vi "Field List Set Default.vi"(6 "FIELD (empty)":T2={"ixField"=0, "iSequenceOrder"=0, "sxFieldId"="", "sxSequenceId"="", "sDisplayName"="", "sValue"="", "sUnits"="", "nDataType"=enum."timestamp", "nNextItem"=enum."Reset", "fSystem"=FALSE, "fSystemValue"=FALSE, "fRequired"=FALSE, "fSetAtTest"=FALSE, "fTestField"=FALSE, "fDeleted"=FALSE, "fIndexed"=FALSE, "fFreeList"=FALSE}, 8 "error in (no error)":errorcluster, 9 "Default Value (\"\")":string, 10 "Flat List (\"\")":string, 11 "Connection Refnum":T1) -> (0 "error out":errorcluster, 2 "New Flat List":string, 3 "dup Connection Refnum":T1)   [LabVIEW 2011]
uses:
  Field Record.ctl
  Field DataTypes.ctl
  Field NextItem.ctl
  Summitek EXT/ODBC/SQL Controls/Connection Refnum.ctl
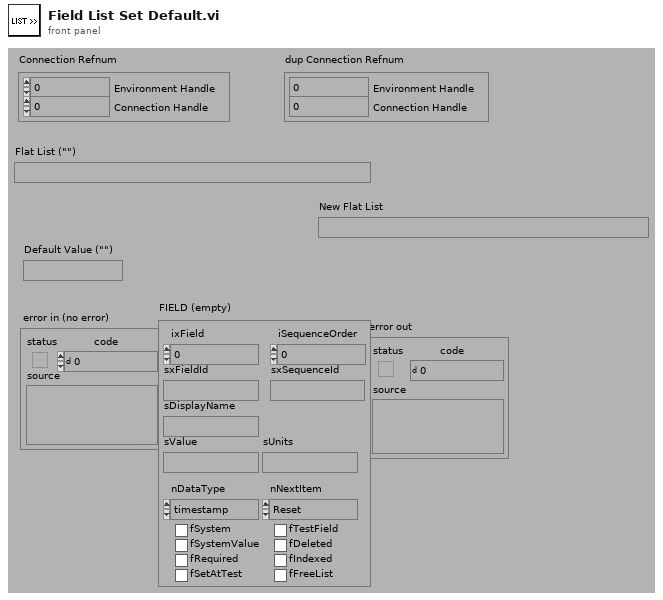
[diagram p1: front panel]
types:
  T1 = typedef "Connection Refnum.ctl" = cluster{"Environment Handle":i32, "Connection Handle":i32}
  T2 = typedef "Field Record.ctl" = cluster{"ixField":i32, "iSequenceOrder":i32, "sxFieldId":string, "sxSequenceId":string, "sDisplayName":string, "sValue":string, "sUnits":string, "nDataType":T3, "nNextItem":T4, "fSystem":bool, "fSystemValue":bool, "fRequired":bool, "fSetAtTest":bool, "fTestField":bool, "fDeleted":bool, "fIndexed":bool, "fFreeList":bool}
  T3 = typedef "Field DataTypes.ctl" = enum32{"text", "numeric", "list", "timestamp", "boolean"}
  T4 = typedef "Field NextItem.ctl" = enum32{"Reset", "Retain", "Auto-Increment"}
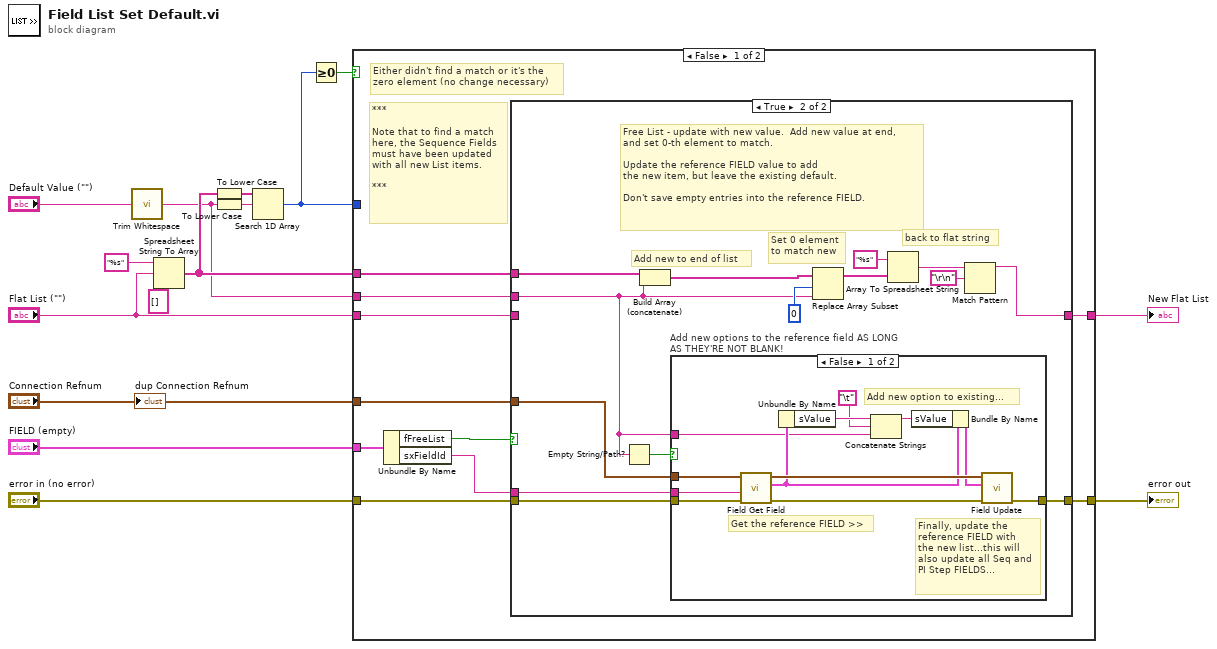
[diagram p0: block diagram]
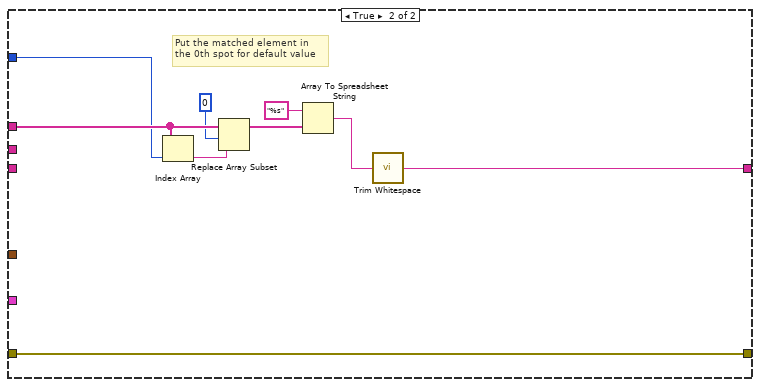
[diagram p4: hidden frame]
diagram:
  n1 = call <vilib>:"Trim Whitespace.vi"("string"="Default Value (\"\")") -> ("trimmed string"=w1:string)  [unwired: 1 in]
  n2 = Spreadsheet String To Array(format string="%s", spreadsheet string="Flat List (\"\")", array type (2D Dbl)=string[] []) -> (array=w7:string[])  [unwired: 1 out]
  n3 = To Lower Case(string=w7) -> (all lower case string=w13:string[])
  n4 = To Lower Case(string=w1) -> (all lower case string=w14:string)
  n5 = Search 1D Array(1D array=w13, element=w14) -> (index of element=w8:i32)  [unwired: 1 out]
  n6 = Greater Or Equal To 0?(x=w8) -> (x >= 0?=w9:bool)
  n7 = case shown="False" w9 {
    tunnel: "Flat List (\"\")" -> [w23 _]
    tunnel: [w22 w56] -> w10
    tunnel: w8 -> [_ w62]
    tunnel: w7 -> [w17 w63]
    tunnel: "Connection Refnum" -> [w20 _]
    tunnel: "FIELD (empty)" -> [w19 _]
    tunnel: "error in (no error)" -> [w25 w55]
    tunnel: [w24 w55] -> w3
    tunnel: w1 -> [w21 _]
    frame False {
      # "***\n\nNote that to find a match\nhere, the Sequence Fields\nmust have been updated\nwith all new List items.\n\n***"
      # "Either didn't find a match or it's the\nzero element (no change necessary)"
      n8 = Unbundle By Name(w19) -> ("fFreeList"=w16:bool, "sxFieldId"=w18:string)
      n9 = case shown="True" w16 {
        tunnel: w25 -> [w26 w40]
        tunnel: [w26 w41] -> w24
        tunnel: w23 -> [w27 _]
        tunnel: [w27 w28] -> w22
        tunnel: w21 -> [_ w32]
        tunnel: w20 -> [_ w39]
        tunnel: w18 -> [_ w38]
        tunnel: w17 -> [_ w36]
        frame False {
          # "Not a Free List - cannot update"
        }
        frame True {
          # "back to flat string"
          # "Set 0 element\nto match new"
          # "Add new to end of list"
          # "Free List - update with new value.  Add new value at end,\nand set 0-th element to match.\n\nUpdate the reference FIELD value to add\nthe new item, but leave the existing default.\n\nDon't save empty entries into the reference FIELD."
          n10 = Empty String/Path?(string/path=w32) -> (empty?=w31:bool)
          n11 = Build Array (concatenate)(w36, w32) -> (w35:string[])
          n12 = case "Add new options to the reference field AS LONG AS THEY'RE NOT BLANK!" shown="False" w31 {
            tunnel: [w53 w54] -> w41
            tunnel: w40 -> [w52 w54]
            tunnel: w39 -> [w50 _]
            tunnel: w38 -> [w47 _]
            tunnel: w32 -> [w42 _]
            frame False {
              # "Add new option to existing..."
              # "Get the reference FIELD >>"
              # "Finally, update the\nreference FIELD with\nthe new list...this will\nalso update all Seq and\nPI Step FIELDS..."
              n13 = call "Field Get Field.vi"("error in (no error)"=w52, "sFieldId or sDisplayName (\"\")"=w47, "Connection Refnum"=w50) -> ("error out"=w51:errorcluster, "Field"=w46:T2, "Connection Refnum"=w49:T1)  [unwired: 2 in, 4 out]
              n14 = Unbundle By Name(w46) -> ("sValue"=w45:string)
              n15 = Concatenate Strings(w45, "\t", w42) -> (w43:string)
              n16 = Bundle By Name(cluster=w46, "sValue"=w43) -> (w48:T2)
              n17 = call "Field Update.vi"("error in (no error)"=w51, "Field Record"=w48, "Connection Refnum"=w49) -> ("error out"=w53:errorcluster)  [unwired: 8 out]
            }
            frame True {
            }
          }
          n18 = Replace Array Subset(array=w35, new element=w32, index=0) -> (w33:string[])
          n19 = Array To Spreadsheet String(array=w33, 3:"%s" ("format string")) -> (spreadsheet string=w29:string)  [unwired: 1 out]
          n20 = Match Pattern(string=w29, regular expression="\r\n") -> (before substring=w28:string)  [unwired: 4 out]
        }
      }
    }
    frame True {
      # "Put the matched element in\nthe 0th spot for default value"
      n21 = Index Array(array=w63, index=w62) -> (element=w60:string)
      n22 = Replace Array Subset(array=w63, new element=w60, index=0) -> (w59:string[])
      n23 = Array To Spreadsheet String(array=w59, 3:"%s" ("format string")) -> (spreadsheet string=w57:string)  [unwired: 1 out]
      n24 = call <vilib>:"Trim Whitespace.vi"("string"=w57) -> ("trimmed string"=w56:string)  [unwired: 1 in]
    }
  }
  "New Flat List" <- w10
  "error out" <- w3
  "dup Connection Refnum" <- "Connection Refnum"
